vi "Pockels sequence gen-lines.vi"(8 "error in (no error)":errorcluster) -> (0 "error out":errorcluster, 1 "Lines in chunk for the trigger period target (ms)":i32, 3 "Ref Scan Cycles":i32)   [LabVIEW 2020]
uses:
  Typedefs/Pockels modulation setup cluster.ctl
  Typedefs/Frame Size.ctl
  Globals/gl_Pockels control globals.vi
panel:
  in  "Use simulation input cluster below":bool
  in  "Input values cluster":T1={"Frame Size"=512, "Fill time (us)"=24.5, "Dwell time (us)"=0.1, "Ref scan dwell time (us)"=0.1, "Lines in ref image"=16, "Pixels in ref image line"=16, "Target time between ref triggers (ms)"=2.0} {"Ref scan dwell time (us)" format="%#_13g"; "Pixels in ref image line" scale=2.0..80.0; "Dwell time (us)" format="%#_13g"; "Fill time (us)" format="%#_13g"; "Target time between ref triggers (ms)" min=0.5 max=10.0 step=0.5 format="%#_13g ms"; "Lines in ref image" scale=2.0..80.0; "Frame Size" items=["100X100"=100, "128X128"=128, "200X200"=200, "256X256"=256, "512X512"=512, "1024x1024"=1024, "2048x2048"=2048]}
  out "Time for ref img line (ms)":dbl
  out "time between reference triggers (ms)":dbl[](array[numeric])
  out "Time for reference image (ms)":dbl
  out "Time for main img line (ms)":dbl
  out "time length of each chunk (ms)":dbl[](array[numeric])
  out "Number of lines in each chunk":i32[](array[numeric]) format="%.0f lines each"
  out "Chunks":i32[](array[numeric]) format="%.0f chunks of"
  out "Adjusted time between ref \ntriggers sent to the FPGA (ms)":dbl format="%#_10g"
  out "Actual resulting time between ref triggers (ms)":dbl format="%#_10g"
  # "INPUTS"
  # "INFORMATION"
  # "Possible combinations resulting in a number of chunks with equal number of lines"
  # "+ Time for ref image"
  # "OUTPUTS"
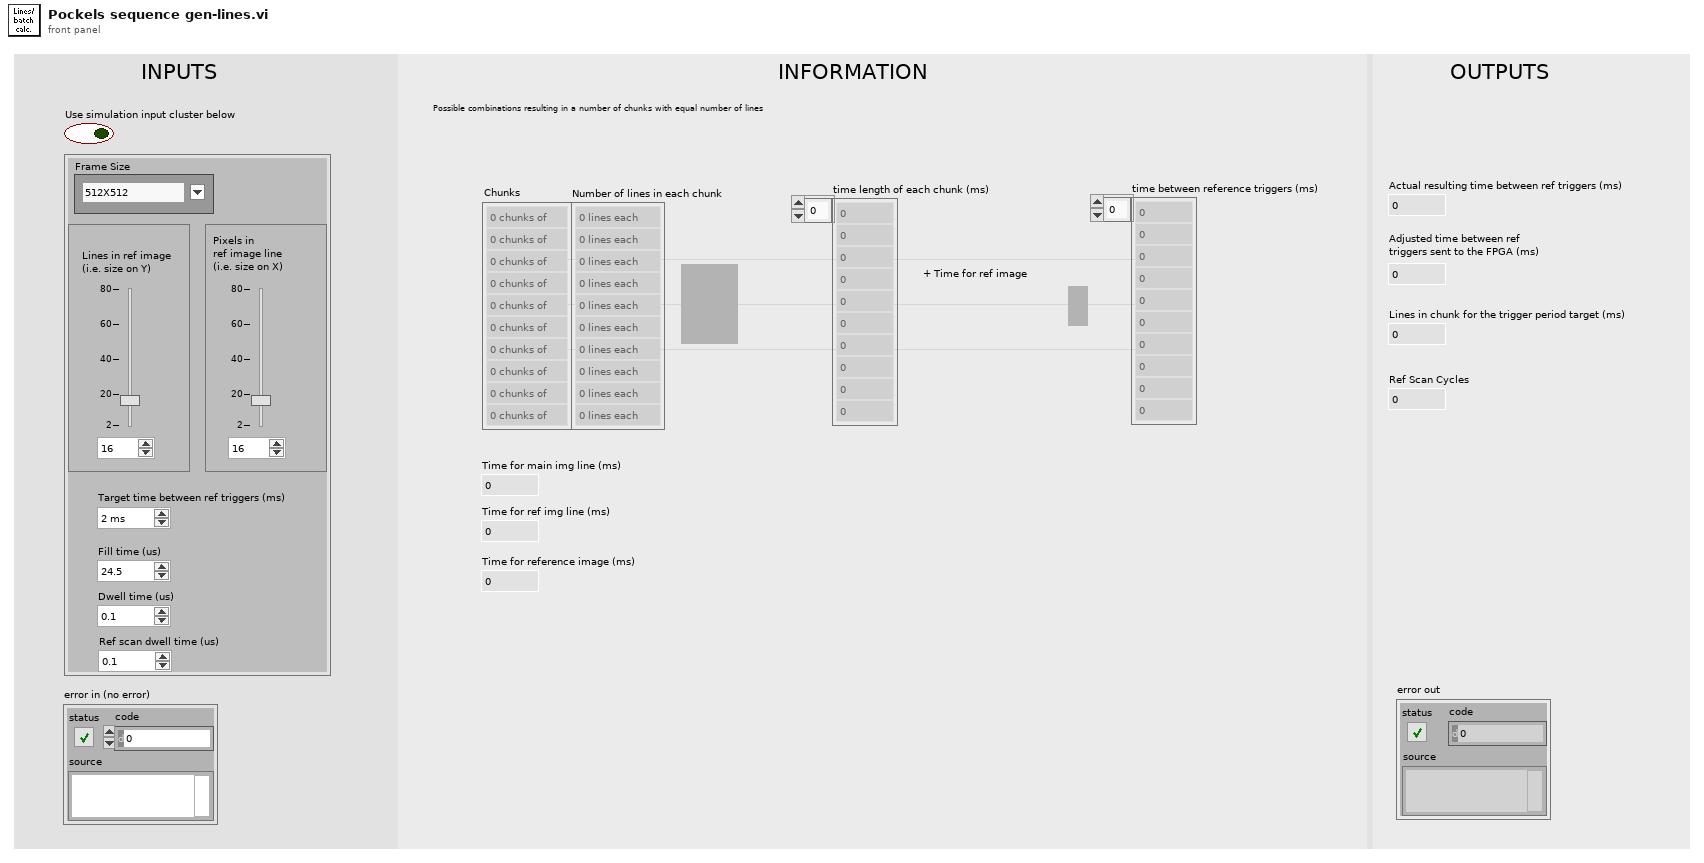
[diagram p1: front panel]
types:
  T1 = typedef "Pockels modulation setup cluster.ctl" = cluster{"Frame Size":T2, "Fill time (us)":dbl, "Dwell time (us)":dbl, "Ref scan dwell time (us)":dbl, "Lines in ref image":i16, "Pixels in ref image line":i16, "Target time between ref triggers (ms)":dbl}
  T2 = typedef "Frame Size.ctl" = u16
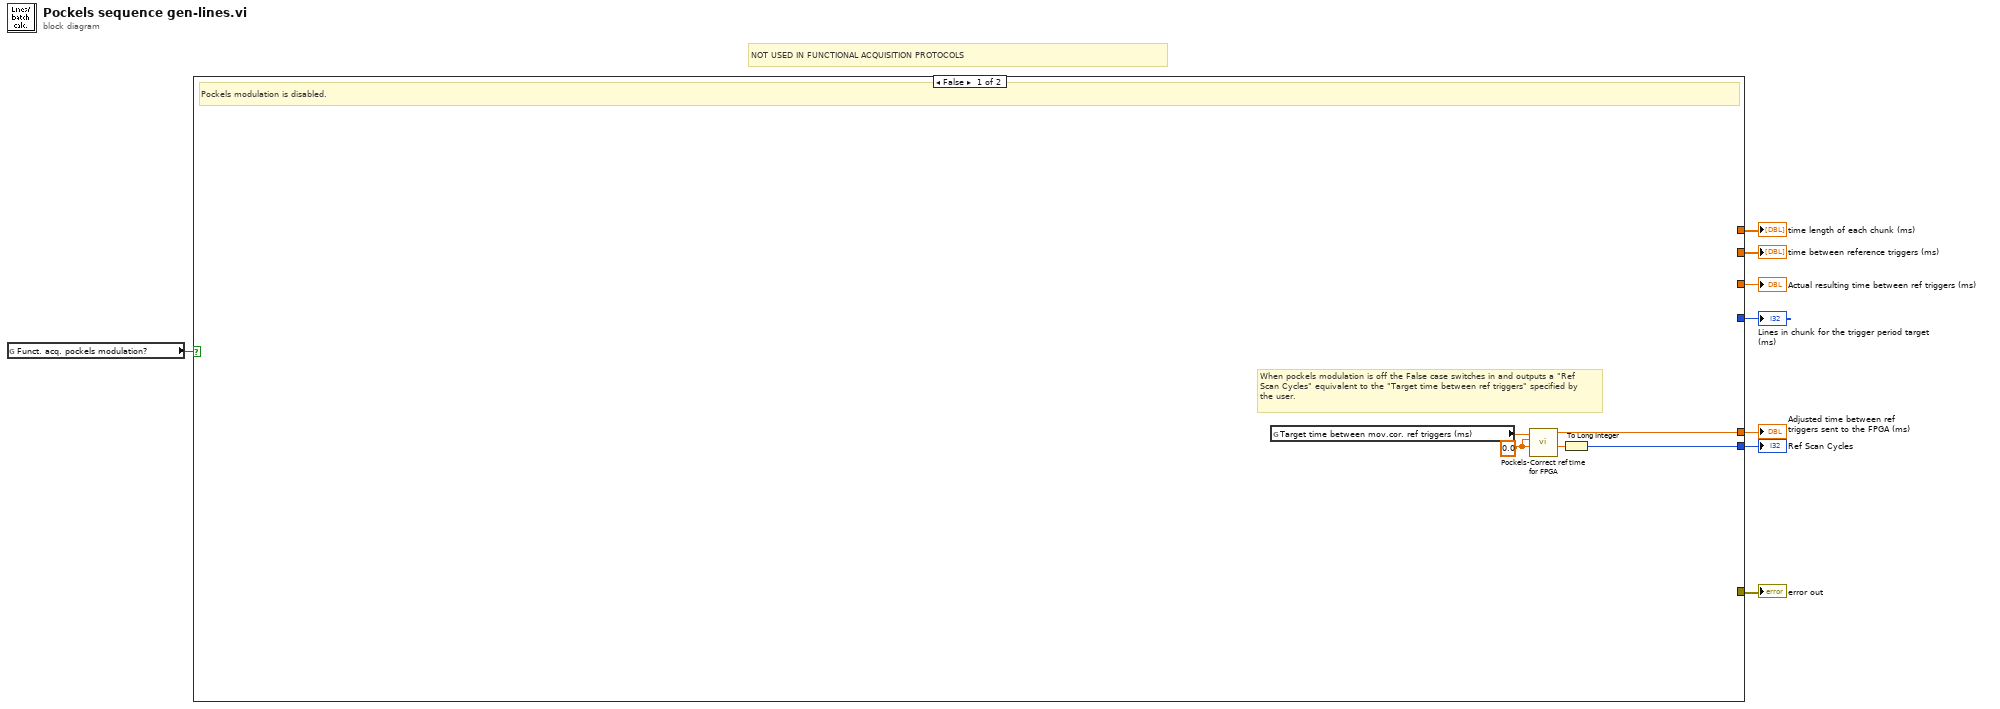
[diagram p0: block diagram]
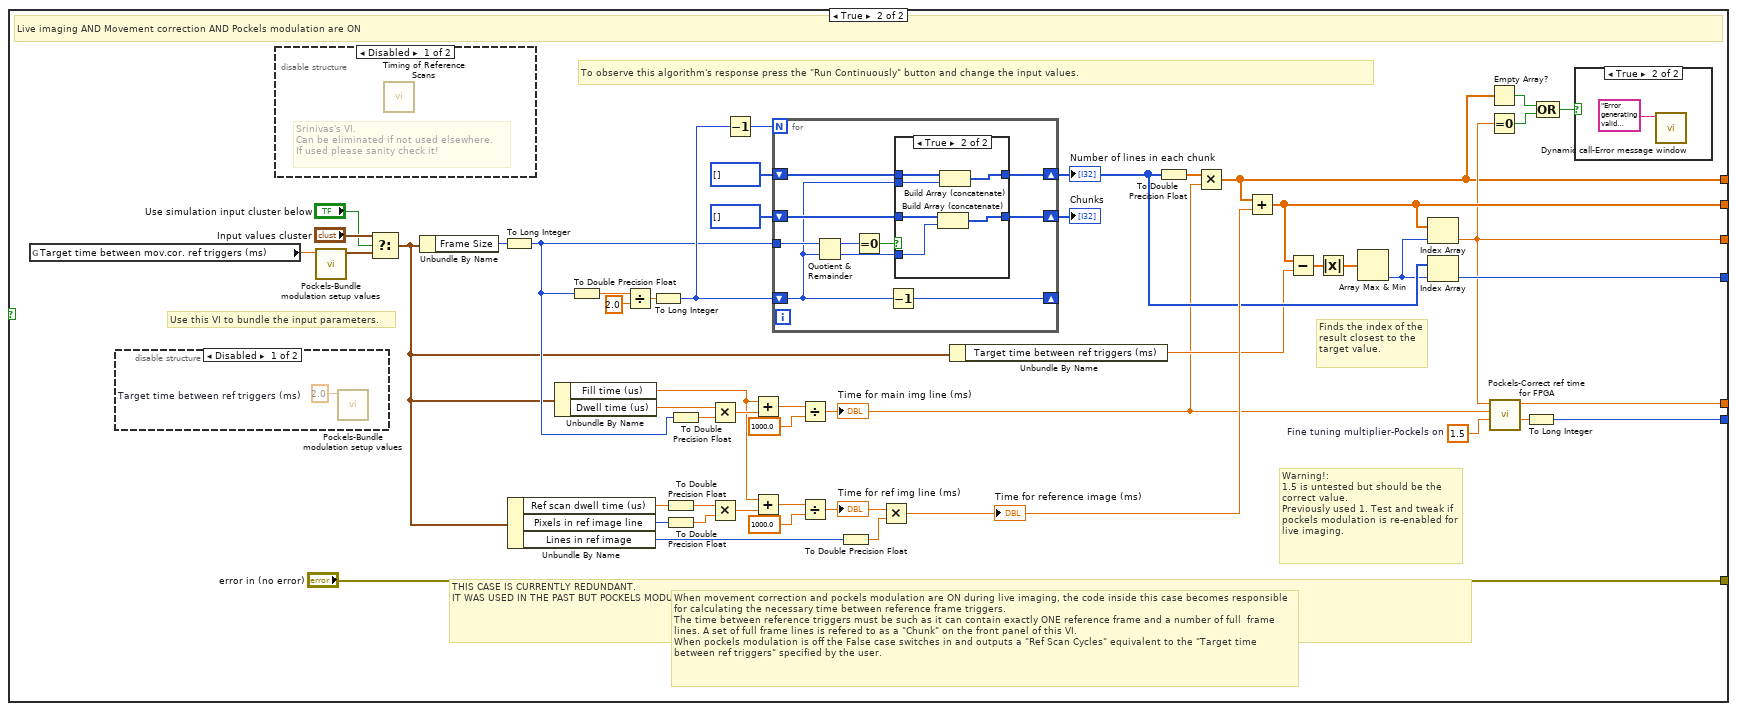
[diagram p2: hidden frame]
diagram:
  # "NOT USED IN FUNCTIONAL ACQUISITION PROTOCOLS"
  n1 = global read "gl_Pockels control globals.vi" "Funct. acq. pockels modulation?"() -> (w1:bool)
  n2 = case shown="False" w1 {
    tunnel: [_ w45] -> w8
    tunnel: [_ w43] -> w7
    tunnel: [w12 w28] -> w6
    tunnel: [w10 w26] -> w5
    tunnel: [_ w20] -> w4
    tunnel: [_ w19] -> w3
    tunnel: [_ "error in (no error)"] -> w2
    frame False {
      w9 = 0.0 ("Time for main img line OR for a single POI (ms)")
      # "When pockels modulation is off the False case switches in and outputs a \"Ref Scan Cycles\" equivalent to the \"Target time between ref triggers\" specified by the user."
      # "Pockels modulation is disabled."
      n3 = global read "gl_Pockels control globals.vi" "Target time between mov.cor. ref triggers (ms)"() -> (w13:dbl)
      n4 = call "Pockels-Correct ref time for FPGA.vi"("Fine tuning multiplier"=w9, "Time for main img line OR for a single POI (ms)"=w9, "Actual resulting time between ref triggers (ms)"=w13) -> ("Ref Scan Cycles"=w11:dbl, "Adjusted time between ref \ntriggers sent to the FPGA (ms)"=w12:dbl)  [unwired: 7 in]
      n5 = To Long Integer(number=w11) -> (32bit integer=w10:i32)
    }
    frame True {
      w14 = 1.5  # Fine tuning multiplier-Pockels on
      # "Warning!:\n1.5 is untested but should be the correct value.\nPreviously used 1. Test and tweak if pockels modulation is re-enabled for live imaging."
      # "THIS CASE IS CURRENTLY REDUNDANT.\nIT WAS USED IN THE PAST BUT POCKELS MODULATION IS NOW KEPT DISABLED FOR LIVE IMAGING"
      # "When movement correction and pockels modulation are ON during live imaging, the code inside this case becomes responsible for calculating the necessary time between reference frame triggers.\nThe time between reference triggers must be such as it can contain exactly ONE reference frame and a number of full  frame lines. A set of full frame lines is refered to as a \"Chunk\" on the front panel of this VI.\nWhen pockels modulation is off the False case switches in and outputs a \"Ref Scan Cycles\" equivalent to the \"Target time between ref triggers\" specified by the user."
      # "Use this VI to bundle the input parameters."
      # "To observe this algorithm's response press the \"Run Continuously\" button and change the input values."
      # "Finds the index of the result closest to the target value."
      # "Live imaging AND Movement correction AND Pockels modulation are ON"
      n6 = global read "gl_Pockels control globals.vi" "Target time between mov.cor. ref triggers (ms)"() -> (w25:dbl)
      n7 = disable-structure "Diagram Disable Structure" shown="Disabled" {
        frame Disabled {
          w66 = 2.0  # Target time between ref triggers (ms)
          n8 = call "Pockels-Bundle modulation setup values.vi"("Target time between ref triggers (ms)"=w66) -> ()  [unwired: 10 in, 1 out]
        }
        frame Enabled {
        }
      }
      n9 = disable-structure "Diagram Disable Structure" shown="Disabled" {
        frame Disabled {
          # "Srinivas's VI.\nCan be eliminated if not used elsewhere.\nIf used please sanity check it!"
          n10 = call "Timing of Reference Scans.vi"() -> ()  [unwired: 9 in, 3 out]
        }
        frame Enabled {
        }
      }
      n11 = call "Pockels-Bundle modulation setup values.vi"("Target time between ref triggers (ms)"=w25) -> ("Pockels modul. setup cluster"=w24:T1)  [unwired: 10 in]
      n12 = Select(t="Input values cluster", s="Use simulation input cluster below", f=w24) -> (s? t:f=w22:T1)
      n13 = Unbundle By Name(w22) -> ("Frame Size"=w39:T2)
      n14 = To Long Integer(number=w39) -> (32bit integer=w41:i32)
      n15 = Unbundle By Name(w22) -> ("Ref scan dwell time (us)"=w31:dbl, "Pixels in ref image line"=w34:i16, "Lines in ref image"=w35:i16)
      n16 = Unbundle By Name(w22) -> ("Fill time (us)"=w37:dbl, "Dwell time (us)"=w33:dbl)
      n17 = To Double Precision Float(number=w41) -> (double precision float=w62:dbl)
      n18 = Divide(x=w62, y=2.0) -> (x/y=w63:dbl)
      n19 = To Long Integer(number=w63) -> (32bit integer=w61:i32)
      n20 = To Double Precision Float(number=w31) -> (double precision float=w30:dbl)
      n21 = To Double Precision Float(number=w34) -> (double precision float=w49:dbl)
      n22 = To Double Precision Float(number=w41) -> (double precision float=w56:dbl)
      n23 = Multiply(x=w33, y=w56) -> (x*y=w55:dbl)
      n24 = Multiply(x=w30, y=w49) -> (x*y=w50:dbl)
      n25 = Decrement(x=w61) -> (x-1=w58:i32)
      n26 = Add(x=w37, y=w55) -> (x+y=w54:dbl)
      n27 = Add(x=w37, y=w50) -> (x+y=w51:dbl)
      n28 = for {
        N: w58 -> [_]
        tunnel: w41 -> [w76]
        shift-right: [w75] -> _
        shift-left: w61 -> [w67]
        shift-right: [w72] -> w59
        shift-left: i32[] [] -> [w71]
        shift-right: [w69] -> w46
        shift-left: i32[] [] -> [w70]
        n29 = Quotient & Remainder(x=w76, y=w67) -> (x-y*floor(x/y)=w68:i32, floor(x/y)=w73:i32)
        n30 = Equal To 0?(x=w68) -> (x = 0?=w74:bool)
        n31 = Decrement(x=w67) -> (x-1=w75:i32)
        n32 = case shown="True" w74 {
          tunnel: w73 -> [_ w84]
          tunnel: [w78 w83] -> w72
          tunnel: w71 -> [w78 w82]
          tunnel: [w77 w80] -> w69
          tunnel: w70 -> [w77 w81]
          tunnel: w67 -> [_ w79]
          frame False {
          }
          frame True {
            n33 = Build Array (concatenate)(w82, w84) -> (w83:i32[])
            n34 = Build Array (concatenate)(w81, w79) -> (w80:i32[])
          }
        }
      }
      "Chunks" <- w59
      "Number of lines in each chunk" <- w46
      n35 = Divide(x=w54, y=1000.0) -> (x/y=w29:dbl)
      "Time for main img line (ms)" <- w29
      n36 = Divide(x=w51, y=1000.0) -> (x/y=w36:dbl)
      "Time for ref img line (ms)" <- w36
      n37 = To Double Precision Float(number=w35) -> (double precision float=w32:dbl)
      n38 = Multiply(x=w36, y=w32) -> (x*y=w48:dbl)
      "Time for reference image (ms)" <- w48
      n39 = Unbundle By Name(w22) -> ("Target time between ref triggers (ms)"=w38:dbl)
      n40 = To Double Precision Float(number=w46) -> (double precision float=w40:dbl[])
      n41 = Multiply(x=w40, y=w29) -> (x*y=w19:dbl[])
      n42 = Add(x=w19, y=w48) -> (x+y=w43:dbl[])
      n43 = Subtract(x=w43, y=w38) -> (x-y=w47:dbl[])
      n44 = Absolute Value(x=w47) -> (abs(x)=w44:dbl[])
      n45 = Array Max & Min(array=w44) -> (min index (indices)=w42:i32)  [unwired: 3 out]
      n46 = Index Array(array=w43, index=w42) -> (element=w20:dbl)
      n47 = Index Array(array=w46, index=w42) -> (element=w45:i32)
      n48 = Empty Array?(array=w19) -> (empty?=w18:bool)
      n49 = Equal To 0?(x=w20) -> (x = 0?=w17:bool)
      n50 = call "Pockels-Correct ref time for FPGA.vi"("Fine tuning multiplier"=w14, "Time for main img line OR for a single POI (ms)"=w29, "Actual resulting time between ref triggers (ms)"=w20) -> ("Ref Scan Cycles"=w27:dbl, "Adjusted time between ref \ntriggers sent to the FPGA (ms)"=w28:dbl)  [unwired: 7 in]
      n51 = To Long Integer(number=w27) -> (32bit integer=w26:i32)
      n52 = Compound Arithmetic op=OR(w18, w17) -> (w16:bool)
      n53 = case shown="True" w16 {
        frame False {
        }
        frame True {
          n54 = call "Dynamic call-Error message window.vi"("Error Message"="Error generating valid movement correction pockels modulation AO sequence.") -> ()  [unwired: 10 in, 1 out]
        }
      }
    }
  }
  "time length of each chunk (ms)" <- w3
  "time between reference triggers (ms)" <- w7
  "Lines in chunk for the trigger period target (ms)" <- w8
  "Actual resulting time between ref triggers (ms)" <- w4
  "Adjusted time between ref \ntriggers sent to the FPGA (ms)" <- w6
  "Ref Scan Cycles" <- w5
  "error out" <- w2
